vi "SbigController.vi"() -> ()   [LabVIEW 2009]
uses:
  Controls/SbigCommand.ctl
panel:
  in  "PROCESS":string="SBIG"
  out "SbigName":string
  in  "SbigData":cluster{"TagName":string, "Serial":string}[](array[cluster])=[{"TagName"="PI1-SBIG", "Serial"="01082913E_"}, {"TagName"="PI2-SBIG", "Serial"="02083139__"}]
  out "SbigControllerState":T1(ring)
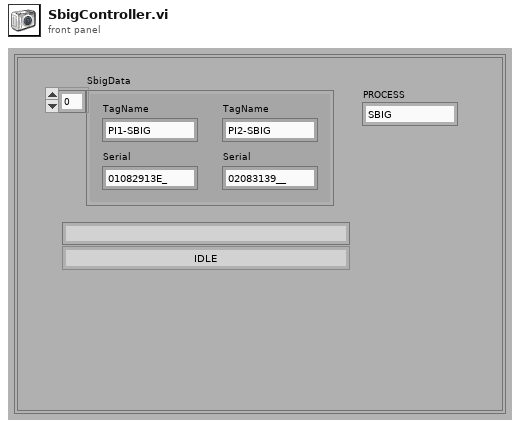
[diagram p1: front panel]
types:
  T1 = enum16{"IDLE", "EXPOSING", "READING", "QUERYING TEMP"}
  T2 = typedef "SbigCommand.ctl" = cluster{"Sbig":string, "Command":enum16{"EXPOSE", "SET TEMP", "SET MISC", "QUIT"}, "Time":u32, "Window":cluster{"X0":u16, "Y0":u16, "DX":u16, "DY":u16, "on/off":bool}, "Temp":cluster{"Regulation":u16, "Auto Freeze":u16, "CCD Set Point":dbl}, "Misc":cluster{"Fan":u16, "Shutter":u16, "Led":u16}}
  T3 = typedef "SbigReference.ctl" = cluster{"Readout modes number":u16, "Readout modes":cluster{"Width":u16, "Height":u16, "Gain":dbl, "pixelWidth":dbl, "pixelHeight":dbl}[], "Handle":u16[]}
  T4 = typedef "SbigCommandQueue.ctl" = refnum<queue>
  T5 = typedef "SbigStatusNotifier.ctl" = refnum<notifier>
  T6 = cluster{"Regulation":u16, "Auto Freeze":u16, "CCD Set Point":dbl}
  T7 = typedef "SbigStatus.ctl" = cluster{"Managed ?":bool, "State":enum16{"IDLE", "EXPOSING", "READING"}, "Image":i32[][], "Temperature Info":cluster{"Temperature Regulation":bool, "T Setpoint":dbl, "T CCD":dbl, "T Ambient":dbl, "Cooling %":dbl}}
  T8 = cluster{"X0":u16, "Y0":u16, "DX":u16, "DY":u16, "on/off":bool}
  T9 = cluster{"Temperature Regulation":bool, "T Setpoint":dbl, "T CCD":dbl, "T Ambient":dbl, "Cooling %":dbl}
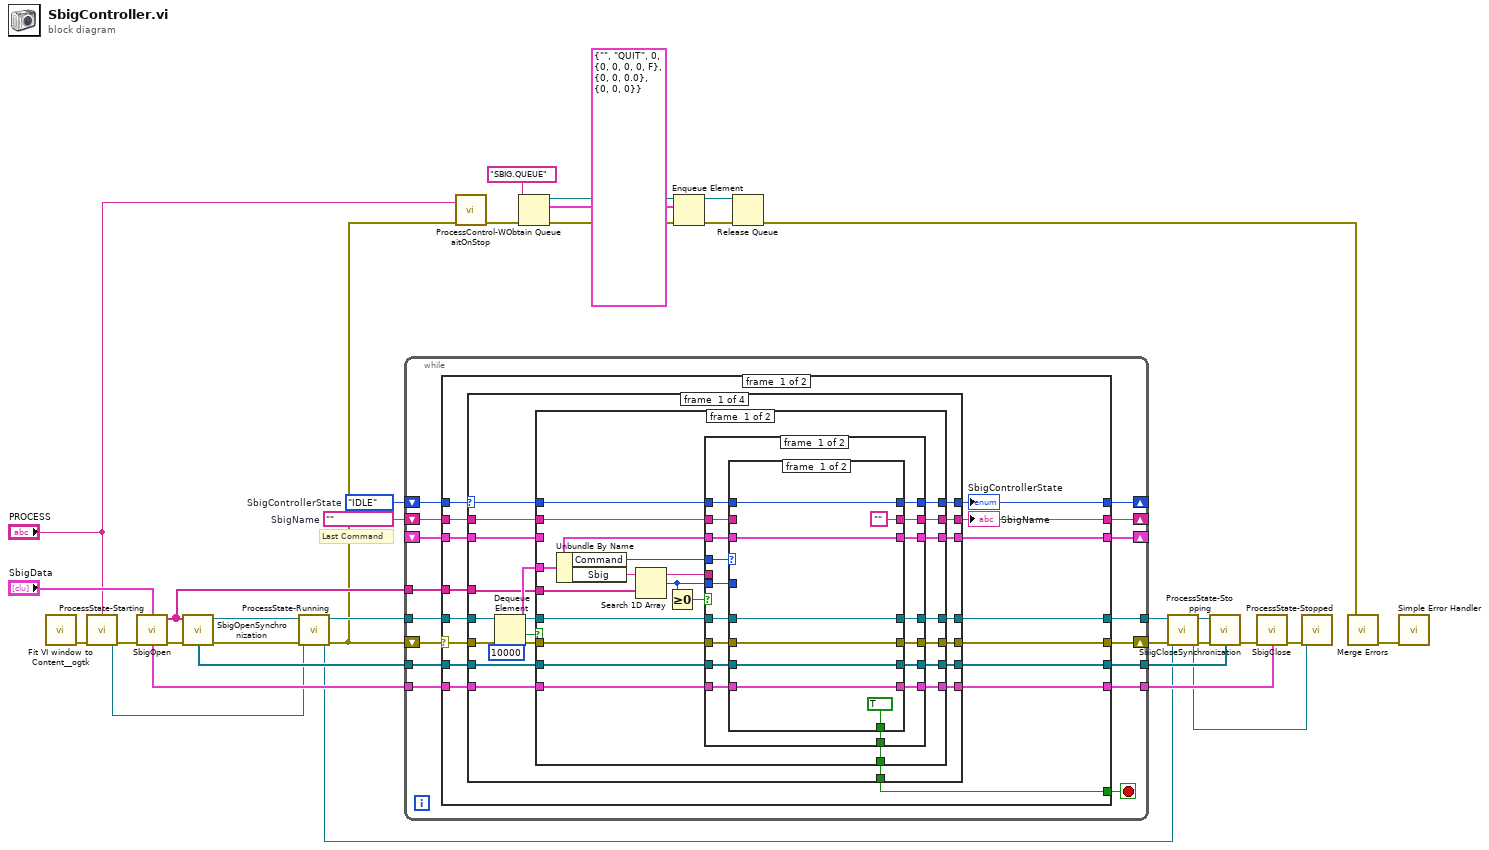
[diagram p0: block diagram]
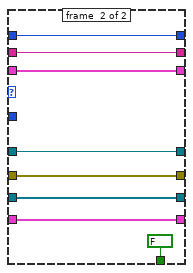
[diagram p2: hidden frame]
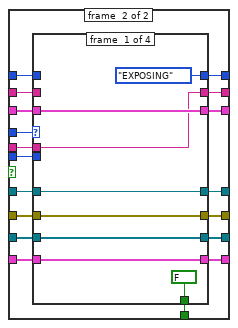
[diagram p3: hidden frame]
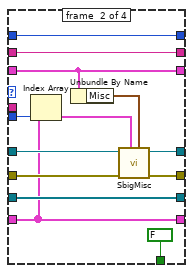
[diagram p4: hidden frame]
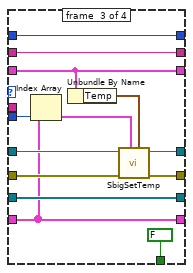
[diagram p5: hidden frame]
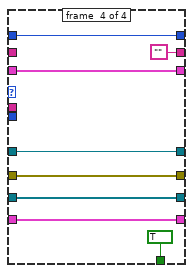
[diagram p6: hidden frame]
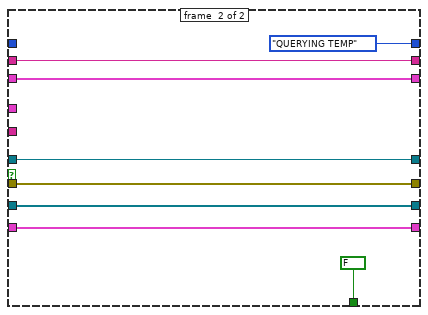
[diagram p7: hidden frame]
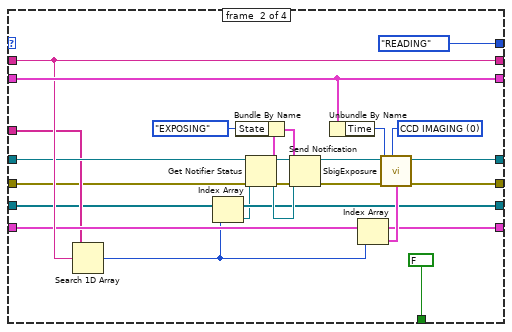
[diagram p8: hidden frame]
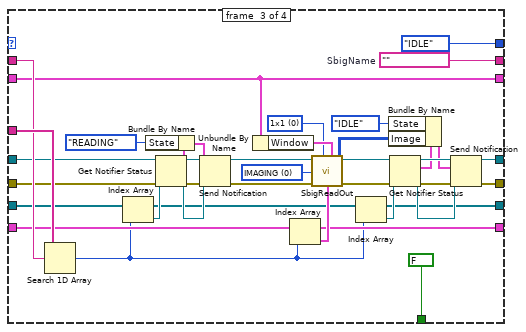
[diagram p9: hidden frame]
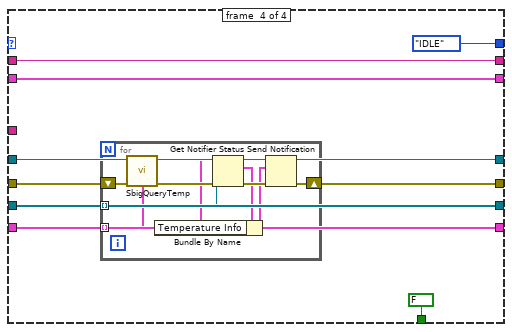
[diagram p10: hidden frame]
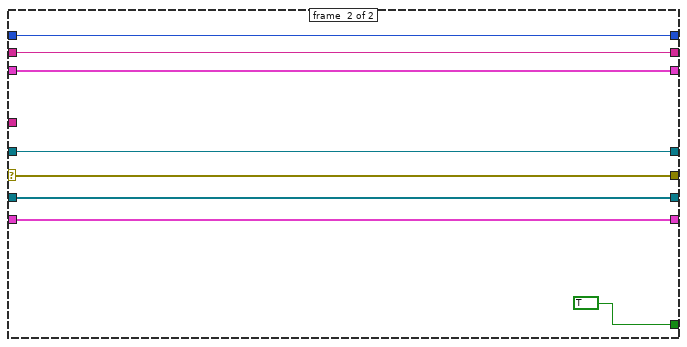
[diagram p11: hidden frame]
diagram:
  w5 = T2 {"Sbig"="", "Command"=enum."QUIT", "Time"=0, "Window"={"X0"=0, "Y0"=0, "DX"=0, "DY"=0, "on/off"=FALSE}, "Temp"={"Regulation"=0, "Auto Freeze"=0, "CCD Set Point"=0.0}, "Misc"={"Fan"=0, "Shutter"=0, "Led"=0}} ("SbigCommand")
  w28 = ""  # SbigName
  w32 = T1."IDLE"  # SbigControllerState
  # "Last Command"
  n1 = call <userlib>:"Fit VI window to Content__ogtk.vi"() -> ("error out"=w18:errorcluster)  [unwired: 3 in, 4 out]
  n2 = call "ProcessState-Starting.vi"("PROCESS"="PROCESS", "error in (no error)"=w18) -> ("ProcessStateNotifier"=w16:refnum<notifier>, "error in (no error)"=w19:errorcluster)  [unwired: 6 out]
  n3 = call "SbigOpen.vi"("SbigDataList"="SbigData", "error in"=w19) -> ("Sbig Names out"=w23:string[], "error out"=w27:errorcluster, "Sbig infos"=w26:T3[])  [unwired: 2 in, 3 out]
  n4 = call "SbigOpenSynchronization.vi"("Sbig List"=w23, "error in (no error)"=w27) -> ("Command Queue out"=w20:T4, "error out"=w17:errorcluster, "Notifiers out"=w30:T5[])  [unwired: 5 out]
  n5 = call "ProcessState-Running.vi"("ProcessStateNotifier in"=w16, "error in (no error)"=w17) -> ("ProcessStateNotifier out"=w13:refnum<notifier>, "error out"=w10:errorcluster)  [unwired: 6 out]
  n6 = while {
    shift-right: [w37] -> _
    shift-left: w32 -> [w48]
    shift-right: [w47] -> w15
    shift-left: w10 -> [w44]
    tunnel: [w45] -> w31
    tunnel: w20 -> [w43]
    tunnel: w30 -> [w42]
    tunnel: [w41] -> w29
    shift-right: [w39] -> _
    shift-left: w28 -> [w40]
    tunnel: w26 -> [w38]
    tunnel: [w36] -> w24
    shift-right: [w35] -> _
    shift-left: _ -> [w34]
    tunnel: w23 -> [w33]
    stop <- w46 stop-if-true
    n7 = case shown="No Error" w44 {
      selector: w44 -> [w63 w281]
      tunnel: w48 -> [w64 w282]
      tunnel: [w55 w281] -> w47
      tunnel: [w54 w282] -> w37
      tunnel: [w59 TRUE] -> w46
      tunnel: [w58 w279] -> w45
      tunnel: w43 -> [w62 w279]
      tunnel: w42 -> [w61 w276]
      tunnel: [w60 w276] -> w41
      tunnel: w40 -> [w57 w278]
      tunnel: [w49 w278] -> w39
      tunnel: w38 -> [w56 w275]
      tunnel: [w53 w275] -> w36
      tunnel: [w52 w277] -> w35
      tunnel: w34 -> [w51 w277]
      tunnel: w33 -> [w50 _]
      frame #0 {
        n8 = case shown="\"QUERYING TEMP\"" w64 {
          selector: w64 -> [w72 _ _ _]
          tunnel: w63 -> [w85 w210 w232 w264]
          tunnel: w62 -> [w84 w217 w245 w256]
          tunnel: [w82 T1."READING" ("SbigControllerState") T1."IDLE" ("SbigControllerState") T1."IDLE" ("SbigControllerState")] -> w54
          tunnel: w61 -> [w81 w207 w229 w262]
          tunnel: [w73 w207 w229 w262] -> w60
          tunnel: [w76 FALSE FALSE FALSE] -> w59
          tunnel: [w75 w217 w245 w256] -> w58
          tunnel: w57 -> [w78 w220 w252 w258]
          tunnel: [w77 w220 w226 w258] -> w49
          tunnel: w56 -> [w70 w218 w249 w261]
          tunnel: [w74 w223 w250 w263] -> w55
          tunnel: [w71 w218 w249 w261] -> w53
          tunnel: [w69 w222 w244 w257] -> w52
          tunnel: w51 -> [w66 w222 w244 w257]
          tunnel: w50 -> [w68 w216 w253 _]
          frame #0 {
            n9 = Dequeue Element(queue=w84, timeout in ms (-1)=10000 ("timeout en ms (-1)"), error in (no error)=w85) -> (queue out=w80:T4, element=w79:T2, timed out?=w67:bool, error out=w83:errorcluster)
            n10 = case shown="True" w67 {
              tunnel: w83 -> [w105 w197]
              tunnel: [w103 T1."QUERYING TEMP" ("SbigControllerState")] -> w82
              tunnel: w81 -> [w102 w200]
              tunnel: w80 -> [w101 w202]
              tunnel: w79 -> [w90 _]
              tunnel: w78 -> [w100 w204]
              tunnel: [w99 w204] -> w77
              tunnel: [w98 FALSE] -> w76
              tunnel: [w97 w202] -> w75
              tunnel: [w96 w197] -> w74
              tunnel: [w95 w200] -> w73
              tunnel: w72 -> [w94 _]
              tunnel: [w93 w199] -> w71
              tunnel: w70 -> [w92 w199]
              tunnel: [w91 w203] -> w69
              tunnel: w68 -> [w87 _]
              tunnel: w66 -> [_ w203]
              frame #0 {
                n11 = Unbundle By Name(w90) -> ("Command"=w104:enum16{"EXPOSE", "SET TEMP", "SET MISC", "QUIT"}, "Sbig"=w86:string)
                n12 = Search 1D Array(1D array=w87, element=w86) -> (index of element=w88:i32)  [unwired: 1 out]
                n13 = Greater Or Equal To 0?(x=w88) -> (x >= 0?=w89:bool)
                n14 = case shown="False" w89 {
                  tunnel: w105 -> [w115 w156]
                  tunnel: w104 -> [w118 w155]
                  tunnel: [w106 w154] -> w103
                  tunnel: w102 -> [w114 w153]
                  tunnel: w101 -> [w116 w152]
                  tunnel: w100 -> [w120 w151]
                  tunnel: [w107 w150] -> w99
                  tunnel: [w122 w149] -> w98
                  tunnel: [w109 w148] -> w97
                  tunnel: [w110 w147] -> w96
                  tunnel: [w111 w146] -> w95
                  tunnel: w94 -> [w121 w145]
                  tunnel: [w112 w144] -> w93
                  tunnel: w92 -> [w113 w143]
                  tunnel: [w108 w142] -> w91
                  tunnel: w90 -> [w119 w141]
                  tunnel: w88 -> [w117 w140]
                  tunnel: w86 -> [_ w139]
                  frame #0 {
                    n15 = case shown="\"QUIT\"" w118 {
                      tunnel: w115 -> [w127 w134]
                      tunnel: [w125 w138] -> w106
                      tunnel: w114 -> [w126 w133]
                      tunnel: w116 -> [w128 w135]
                      tunnel: w119 -> [w123 w136]
                      tunnel: w120 -> [_ w137]
                      tunnel: ["" ("Sbig") w137] -> w107
                      tunnel: [TRUE FALSE] -> w122
                      tunnel: [w128 w135] -> w109
                      tunnel: [w127 w134] -> w110
                      tunnel: [w126 w133] -> w111
                      tunnel: w121 -> [w125 w138]
                      tunnel: [w124 w132] -> w112
                      tunnel: w113 -> [w124 w132]
                      tunnel: [w123 w136] -> w108
                      tunnel: w117 -> [_ _]
                      frame #0 {
                      }
                      frame #1 {
                      }
                    }
                  }
                  frame #1 {
                    n16 = case shown="\"QUIT\"" w155 {
                      tunnel: w156 -> [w161 w173 w185 w193]
                      tunnel: [T1."EXPOSING" ("SbigControllerState") w175 w187 w191] -> w154
                      tunnel: w153 -> [w160 w170 w182 w192]
                      tunnel: w152 -> [w162 w171 w183 w194]
                      tunnel: w141 -> [w159 w168 w180 w189]
                      tunnel: w151 -> [_ w174 w186 _]
                      tunnel: [w157 w174 w186 "" ("Sbig")] -> w150
                      tunnel: [FALSE FALSE FALSE TRUE] -> w149
                      tunnel: [w162 w171 w183 w194] -> w148
                      tunnel: [w161 w172 w184 w193] -> w147
                      tunnel: [w160 w170 w182 w192] -> w146
                      tunnel: w145 -> [_ w175 w187 w191]
                      tunnel: [w163 w169 w181 w190] -> w144
                      tunnel: w143 -> [w163 w169 w181 w190]
                      tunnel: [w159 w168 w180 w189] -> w142
                      tunnel: w140 -> [_ w166 w179 _]
                      tunnel: w139 -> [w157 _ _ _]
                      frame #0 {
                      }
                      frame #1 {
                        n17 = Index Array(array=w169, index=w166) -> (element=w165:T3)
                        n18 = Unbundle By Name(w168) -> ("Misc"=w167:cluster{"Fan":u16, "Shutter":u16, "Led":u16})
                        n19 = call "SbigMisc.vi"("Misc"=w167, "SbigReference"=w165, "error in (no error)"=w173) -> ("error out"=w172:errorcluster)  [unwired: 6 out]
                      }
                      frame #2 {
                        n20 = Index Array(array=w181, index=w179) -> (element=w177:T3)
                        n21 = Unbundle By Name(w180) -> ("Temp"=w178:T6)
                        n22 = call "SbigSetTemp.vi"("Temp Regulation"=w178, "SbigReference"=w177, "error in (no error)"=w185) -> ("error out"=w184:errorcluster)  [unwired: 1 in, 5 out]
                      }
                      frame #3 {
                      }
                    }
                  }
                }
              }
              frame #1 {
              }
            }
          }
          frame #1 {
            w215 = u16 0 items=["CCD IMAGING", "CCD TRACKING"] ("CCD")
            n23 = Search 1D Array(1D array=w216, element=w220) -> (index of element=w205:i32)  [unwired: 1 out]
            n24 = Index Array(array=w207, index=w205) -> (element=w206:T5)
            n25 = Get Notifier Status(notifier=w206, error in (no error)=w210) -> (notifier out=w213:T5, current notification=w212:T7, error out=w214:errorcluster)  [unwired: 2 out]
            n26 = Bundle By Name(cluster=w212, "State"=enum16{"IDLE", "EXPOSING", "READING"}."EXPOSING") -> (w208:T7)
            n27 = Send Notification(notification=w208, notifier=w213, error in (no error)=w214) -> (error out=w209:errorcluster)  [unwired: 1 out]
            n28 = Unbundle By Name(w222) -> ("Time"=w221:u32)
            n29 = Index Array(array=w218, index=w205) -> (element=w219:T3)
            n30 = call "SbigExposure.vi"("error in (no error)"=w209, "Sbig"=w219, "Exposure Time (10ms)"=w221, "CCD"=w215) -> ("error out"=w223:errorcluster)  [unwired: 2 in, 2 out]
          }
          frame #2 {
            w246 = u16 0 items=["1x1", "2x2", "3x3"] ("Binning Mode")
            w227 = u16 0 items=["IMAGING", "TRACKING"] ("CCD")
            w226 = ""  # SbigName
            n31 = Search 1D Array(1D array=w253, element=w252) -> (index of element=w230:i32)  [unwired: 1 out]
            n32 = Index Array(array=w229, index=w230) -> (element=w233:T5)
            n33 = Get Notifier Status(notifier=w233, error in (no error)=w232) -> (notifier out=w237:T5, current notification=w236:T7, error out=w238:errorcluster)  [unwired: 2 out]
            n34 = Bundle By Name(cluster=w236, "State"=enum16{"IDLE", "EXPOSING", "READING"}."READING") -> (w234:T7)
            n35 = Send Notification(notification=w234, notifier=w237, error in (no error)=w238) -> (error out=w231:errorcluster)  [unwired: 1 out]
            n36 = Unbundle By Name(w244) -> ("Window"=w247:T8)
            n37 = Index Array(array=w249, index=w230) -> (element=w251:T3)
            n38 = call "SbigReadOut.vi"("error in (no error)"=w231, "Sbig"=w251, "CCD"=w227, "Binning Mode"=w246, "Window"=w247) -> ("error out"=w243:errorcluster, "Image"=w248:i32[][])  [unwired: 2 out]
            n39 = Index Array(array=w229, index=w230) -> (element=w242:T5)
            n40 = Get Notifier Status(notifier=w242, error in (no error)=w243) -> (notifier out=w241:T5, current notification=w240:T7)  [unwired: 3 out]
            n41 = Bundle By Name(cluster=w240, "State"=enum16{"IDLE", "EXPOSING", "READING"}."IDLE", "Image"=w248) -> (w239:T7)
            n42 = Send Notification(notification=w239, notifier=w241, error in (no error)=w243) -> (error out=w250:errorcluster)  [unwired: 1 out]
          }
          frame #3 {
            n43 = for {
              shift-right: [w270] -> w263
              shift-left: w264 -> [w274]
              tunnel: w261 -> [w273] mode=indexing
              tunnel: w262 -> [w271] mode=indexing
              n44 = call "SbigQueryTemp.vi"("SbigReference"=w273, "error in (no error)"=w274) -> ("Temperature Info"=w265:T9, "error out"=w272:errorcluster)  [unwired: 6 out]
              n45 = Get Notifier Status(notifier=w271, error in (no error)=w272) -> (notifier out=w269:T5, current notification=w267:T7, error out=w268:errorcluster)  [unwired: 2 out]
              n46 = Bundle By Name(cluster=w267, "Temperature Info"=w265) -> (w266:T7)
              n47 = Send Notification(notification=w266, notifier=w269, error in (no error)=w268) -> (error out=w270:errorcluster)  [unwired: 1 out]
            }
          }
        }
        "SbigName" <- w49
        "SbigControllerState" <- w54
      }
      frame #1 {
      }
    }
  }
  n48 = call "ProcessControl-WaitOnStop.vi"("PROCESS"="PROCESS", "error out"=w10) -> ("error in"=w8:errorcluster)  [unwired: 7 out]
  n49 = Obtain Queue(name (unnamed)="SBIG.QUEUE" ("nom (aucun)"), element data type=w5, error in (no error)=w8) -> (queue out=w6:refnum<queue>, error out=w7:errorcluster)  [unwired: 2 in, 1 out]
  n50 = Enqueue Element(queue=w6, element=w5, error in (no error)=w7) -> (queue out=w2:refnum<queue>, error out=w3:errorcluster)  [unwired: 2 out]
  n51 = Release Queue(queue=w2, error in (no error)=w3) -> (error out=w1:errorcluster)  [unwired: 3 out]
  n52 = call "ProcessState-Stopping.vi"("ProcessStateNotifier in"=w13, "error in (no error)"=w15) -> ("ProcessStateNotifier out"=w11:refnum<notifier>, "error out"=w14:errorcluster)  [unwired: 6 out]
  n53 = call "SbigCloseSynchronization.vi"("Queue in"=w31, "Notifiers in"=w29, "error in (no error)"=w14) -> ("error out (no error)"=w25:errorcluster)  [unwired: 1 in, 5 out]
  n54 = call "SbigClose.vi"("error in"=w25, "Sbig infos"=w24) -> ("error out"=w12:errorcluster)  [unwired: 3 out]
  n55 = call "ProcessState-Stopped.vi"("ProcessStateNotifier in"=w11, "error in (no error)"=w12) -> ()  [unwired: 8 out]
  n56 = call <vilib>:"Merge Errors.vi"("error in 1 (no error)"=w1) -> ("error out"=w21:errorcluster)  [unwired: 3 in, 3 out]
  n57 = call <vilib>:"Simple Error Handler.vi"("error in (no error)"=w21) -> ()  [unwired: 1 in, 8 out]
